vi "Add RequirementID.vi"(7 "overwrite?":bool=TRUE, 9 "error in (no error)":errorcluster, 10 "Requirement ID":string, 11 "Properties":refnum<class "Properties.lvclass">) -> (1 "error out":errorcluster, 3 "Properties":refnum<class "Properties.lvclass">)   [LabVIEW 2020, in "Caraya.lvlib" / "Properties.lvclass"]
uses:
  Properties.lvclass
  Properties.lvclass/Properties.ctl
  Test Manager Message KVP/TestManagerMsg.KVP.lvclass
  Caraya.lvlib
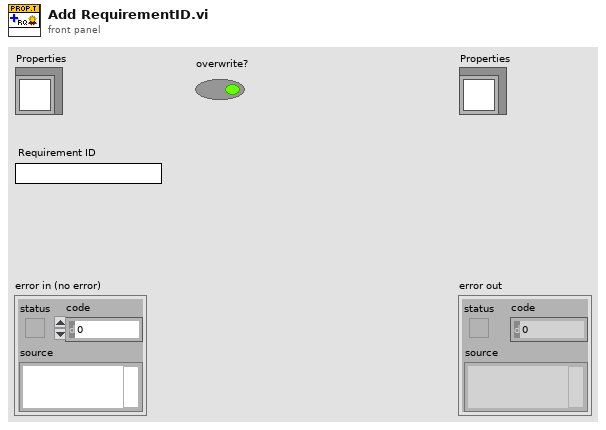
[diagram p1: front panel]
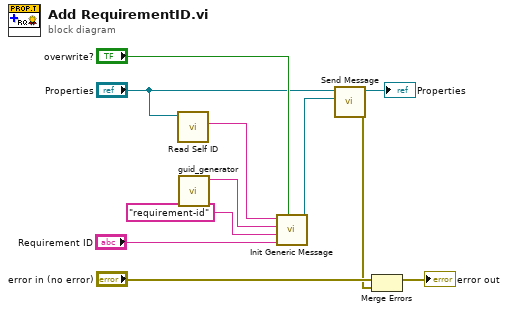
[diagram p0: block diagram]
diagram:
  n1 = call "Read Self ID.vi"("Properties in"="Properties") -> ("self-id"=w2:string)  [unwired: 9 in, 1 out]
  n2 = call "guid_generator.vi"() -> ("guid"=w1:string)  [unwired: 11 in]
  n3 = call "Init Generic Message.vi"("overwrite?"="overwrite?", "value"="Requirement ID", "key"="requirement-id", "self-id"=w1, "owner-id"=w2) -> ("Message"=w3:refnum<class "TestManagerMsg.lvclass">)  [unwired: 6 in]
  n4 = call "Send Message.vi"("TestManagerMsg"=w3, "Properties in"="Properties") -> ("error out"=w4:errorcluster, "Properties out"=→"Properties":refnum<class "Properties.lvclass">)  [unwired: 8 in]
  n5 = Merge Errors("error in (no error)", w4) -> (→"error out":errorcluster)
